vi "test-VAttributes-VAttributesToData(Cluster).vi"(8 "error in (no error)":errorcluster, 11 "TestCase in":refnum<class "MyTestCase.lvclass">) -> (0 "error out":errorcluster, 3 "TestCase out":refnum<class "MyTestCase.lvclass">)   [LabVIEW 2019, in "MyTestCase.lvclass"]
uses:
  MyTestCase.lvclass
  <userlib>/_OpenG.lib/lvdata/lvdata.llb/Type Descriptor Enumeration__ogtk.ctl
  <vilib>/addons/_JKI Toolkits/VI Tester/TestCase.llb/TestCase.lvclass
  lv-apt-json-file.lvlib
  C:/Program Files (x86)/National Instruments/LabVIEW 2019/vi.lib/addons/_JKI Toolkits/VI Tester/TestCase.llb/TestCase.lvclass
panel:
  out "data 5":variant
  out "data 3":variant
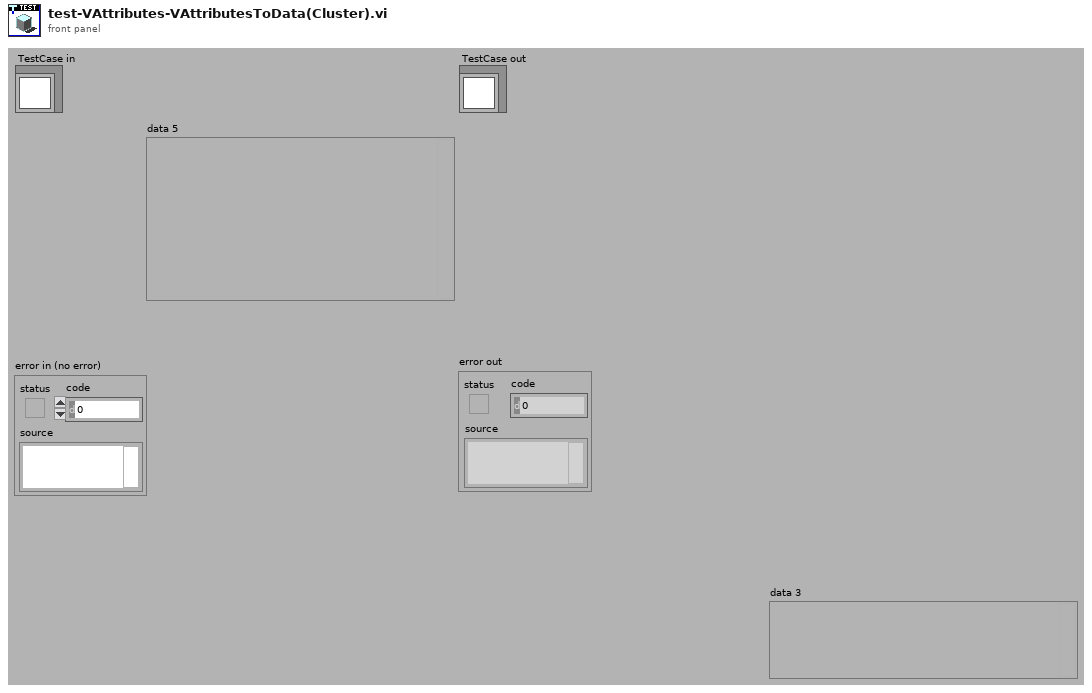
[diagram p1: front panel]
types:
  T1 = typedef "Type Descriptor Enumeration__ogtk.ctl" = enum8{"<Null>", "I8", "I16", "I32", "I64", "U8", "U16", "U32", "U64", "SGL", "DBL", "EXT", "CSG", "CDB", "CXT", "0x0F", "0x10", "0x11", "0x12", "0x13", "0x14", "Enum U8", "Enum U16", "Enum U32", "Enum U64", "SGL PQ", "DBL PQ", "EXT PQ", "CSG PQ", "CDB PQ", "CXT PQ", "0x1F", "0x20", "Boolean", "0x22", "0x23", "0x24", "0x25", "0x26", "0x27", "0x28", "0x29", "0x2A", "0x2B", "0x2C", "0x2D", "0x2E", "0x2F", "String", "0x31", "Path", "Pict", "0x34", "0x35", "0x36", "DAQ", "0x38", "0x39", "0x3A", "0x3B", "0x3C", "0x3D", "0x3E", "0x3F", "Array", "0x41", "0x42", "0x43", "0x44", "0x45", "0x46", "0x47", "0x48", "0x49", "0x4A", "0x4B", "0x4C", "0x4D", "0x4E", "0x4F", "Cluster", "0x51", "0x52", "Variant", "Waveform", "0x55", "0x56", "0x57", "0x58", "0x59", "0x5A", "0x5B", "0x5C", "0x5D", "0x5E", "Fixed Point", "0x60", "0x61", "0x62", "0x63", "0x64", "0x65", "0x66", "0x67", "0x68", "0x69", "0x6A", "0x6B", "0x6C", "0x6D", "0x6E", "0x6F", "Refnum", "0x71", "0x72", "Set Collection", "Map Collection"}
  T2 = cluster{"numeric":i32, "string":string, "Cluster":cluster{"numeric":i32, "string":string, "cluster":cluster{"numeric":i32, "string":string, "cluster":cluster{"numeric":i32, "string":string}}}}
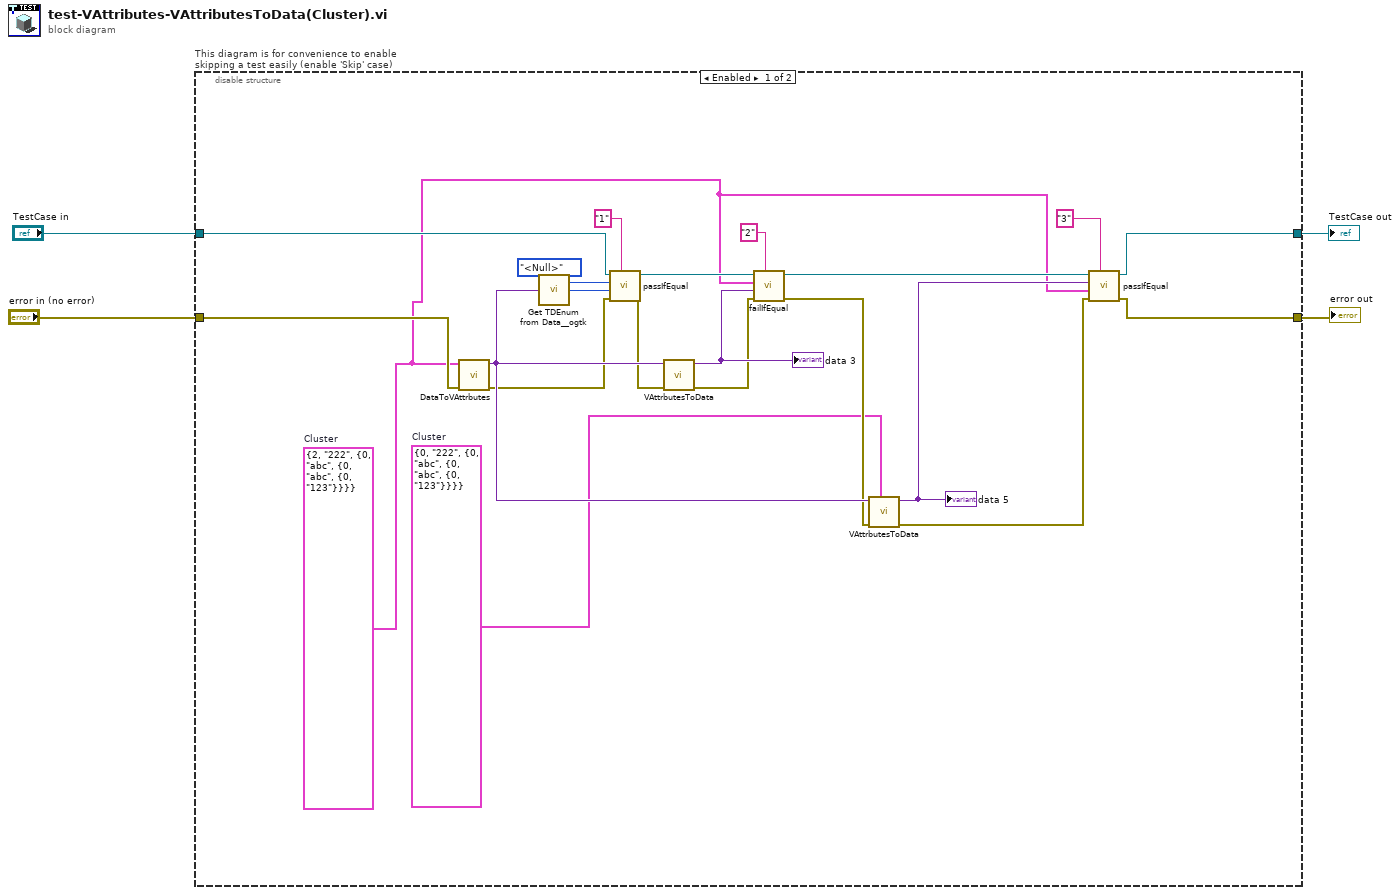
[diagram p0: block diagram]
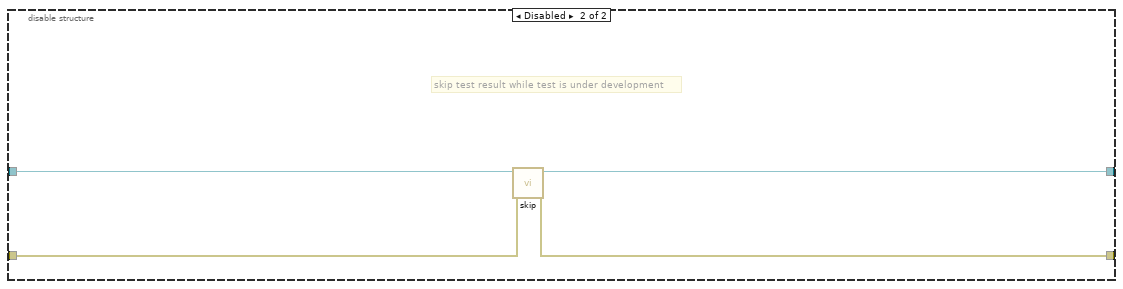
[diagram p2: hidden frame]
diagram:
  n1 = disable-structure "This diagram is for convenience to enable skipping a test easily (enable 'Skip' case)" shown="Enabled" {
    disable-tunnel: "TestCase in" -> [w24 w29]
    disable-tunnel: [w18 w27] -> w1
    disable-tunnel: [w12 w28] -> w3
    disable-tunnel: "error in (no error)" -> [w25 w26]
    frame Enabled {
      w6 = T2 {"numeric"=0, "string"="222", "Cluster"={"numeric"=0, "string"="abc", "cluster"={"numeric"=0, "string"="abc", "cluster"={"numeric"=0, "string"="123"}}}}  # Cluster
      w5 = T2 {"numeric"=2, "string"="222", "Cluster"={"numeric"=0, "string"="abc", "cluster"={"numeric"=0, "string"="abc", "cluster"={"numeric"=0, "string"="123"}}}}  # Cluster
      n2 = call "DataToVAttrbutes.vi"("error in (no error)"=w25, "data"=w5) -> ("error out"=w17:errorcluster, "VAttributes"=w19:variant)  [unwired: 8 in]
      n3 = call <userlib>:"Get TDEnum from Data__ogtk.vi"("Data"=w19) -> ("Type Descriptor Enumeration"=w11:T1)  [unwired: 4 in]
      n4 = call-dynamic "passIfEqual.vi"("custom report message (\"\")"="1" ("custom report message (\"\")"), "error in (no error)"=w17, "y"=w11, "x"=Type_Descriptor_Enumeration__ogtk."<Null>" ("Type Descriptor Enumeration"), "TestCase in"=w24) -> ("error out"=w16:errorcluster, "TestCase out"=w22:refnum<class "MyTestCase.lvclass">)  [unwired: 5 in]
      n5 = call "VAttrbutesToData.vi"("error in (no error)"=w16, "VAttributes"=w19) -> ("error out"=w15:errorcluster, "data"=w23:variant)  [unwired: 8 in]
      "data 3" <- w23
      n6 = call-dynamic "failIfEqual.vi"("custom report message (\"\")"="2" ("custom report message (\"\")"), "error in (no error)"=w15, "y"=w23, "x"=w5, "TestCase in"=w22) -> ("error out"=w14:errorcluster, "TestCase out"=w21:refnum<class "MyTestCase.lvclass">)  [unwired: 5 in]
      n7 = call "VAttrbutesToData.vi"("Prototype"=w6, "error in (no error)"=w14, "VAttributes"=w19) -> ("error out"=w13:errorcluster, "data"=w20:variant)  [unwired: 7 in]
      "data 5" <- w20
      n8 = call-dynamic "passIfEqual.vi"("custom report message (\"\")"="3" ("custom report message (\"\")"), "error in (no error)"=w13, "y"=w5, "x"=w20, "TestCase in"=w21) -> ("error out"=w12:errorcluster, "TestCase out"=w18:refnum<class "MyTestCase.lvclass">)  [unwired: 5 in]
    }
    frame Disabled {
      # "skip test result while test is under development"
      n9 = call <vilib>:"skip.vi"("error in (no error)"=w26, "TestCase in"=w29) -> ("error out"=w28:errorcluster, "TestCase out"=w27:refnum<class "MyTestCase.lvclass">)  [unwired: 8 in]
    }
  }
  "error out" <- w3
  "TestCase out" <- w1
